vi "Init Hardware.vi"(8 "error in (no error)":errorcluster, 11 "Tektronix Driver in":refnum<class "Tektronix 4000 Driver.lvclass">) -> (0 "error out":errorcluster, 3 "Tektronix Driver out":refnum<class "Tektronix 4000 Driver.lvclass">)   [LabVIEW 2020, in "Tektronix 4000 Driver.lvclass"]
uses:
  Tektronix 4000 Driver.lvclass
  C:/GitHub/NHMFL_Core/Libraries/Instruments/Tektronix/Tektronix Driver/Tektronix Driver.lvclass
  <instrlib>/Tektronix DPO MSO 2000 4000 Series/Tektronix DPO MSO 2000 4000 Series.lvlib
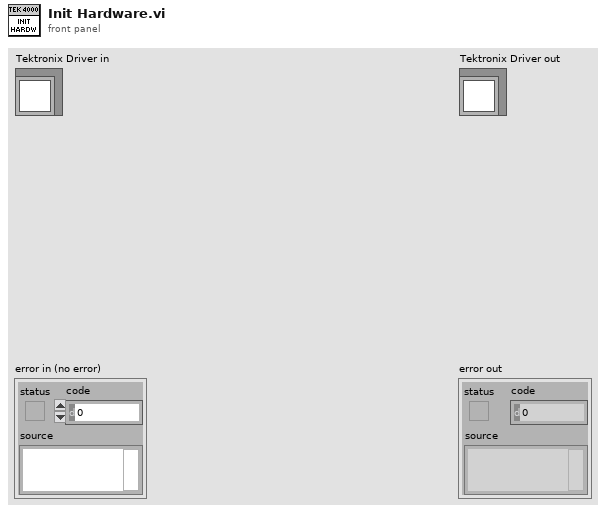
[diagram p1: front panel]
types:
  T1 = typedef "Tektronix Configuration.ctl" = cluster{"Channel":i32, "Number of averages":i32, "Input impedace":enum16{"1 M Ohm", "50 Ohm"}, "Vertical coupling":enum16{"AC", "DC", "Ground"}}
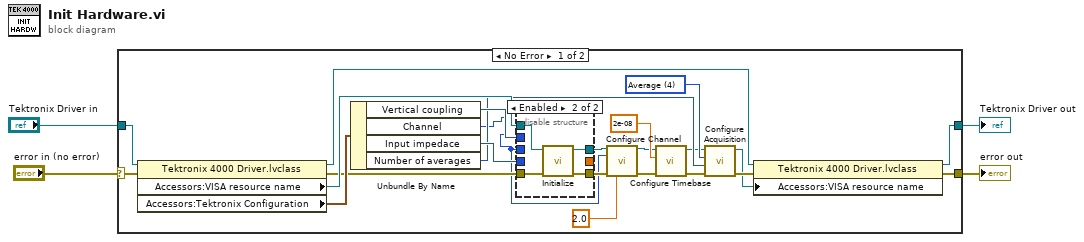
[diagram p0: block diagram]
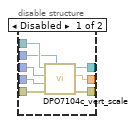
[diagram p2: hidden frame]
diagram:
  n1 = case shown="No Error" "error in (no error)" {
    selector: "error in (no error)" -> [w27 w41]
    tunnel: [w20 w41] -> w3
    tunnel: [w18 w40] -> w1
    tunnel: "Tektronix Driver in" -> [w26 w40]
    frame No Error {
      w17 = u16 4 items=["Sample", "Peak Detect", "Hi Res", "Envelope", "Average"] ("Acquisition Type (0: Sample)")
      n2 = property class="Tektronix 4000 Driver.lvclass"(reference=w26, error in=w27) -> (reference out=w19:refnum<class "Tektronix 4000 Driver.lvclass">, error out=w23:errorcluster, "Accessors:VISA resource name"=w25:refnum<visa-resource-name>, "Accessors:Tektronix Configuration"=w24:T1)
      n3 = Unbundle By Name(w24) -> ("Vertical coupling"=w22:enum16{"AC", "DC", "Ground"}, "Channel"=w6:i32, "Input impedace"=w21:enum16{"1 M Ohm", "50 Ohm"}, "Number of averages"=w16:i32)
      n4 = disable-structure shown="Enabled" {
        disable-tunnel: w25 -> [w35 w39]
        disable-tunnel: w23 -> [w34 w38]
        disable-tunnel: w22 -> [w33 _]
        disable-tunnel: [w32 _] -> _
        disable-tunnel: [w31 w36] -> w7
        disable-tunnel: [w30 w37] -> w10
        disable-tunnel: w6 -> [w29 _]
        disable-tunnel: w21 -> [w28 _]
        frame Disabled {
          n5 = call "DPO7104c_vert_scale.vi"("Vertical Coupling (1: DC)"=w33, "error in (no error)"=w34, "Input Impedance (0: 1M ohm)"=w28, "Channel (0: Channel 1)"=w29, "VISA resource name"=w35) -> ("error out"=w31:errorcluster, "vertical range"=w32:dbl, "VISA resource name out"=w30:refnum<visa-resource-name>)  [unwired: 4 in]
        }
        frame Enabled {
          n6 = call <instrlib>:"Initialize.vi"("error in (no error)"=w38, "VISA resource name"=w39) -> ("error out"=w36:errorcluster, "VISA resource name out"=w37:refnum<visa-resource-name>)  [unwired: 8 in]
        }
      }
      n7 = call <instrlib>:"Configure Channel.vi"("VISA resource name"=w10, "Channel (0: Channel 1)"=w6, "error in (no error)"=w7, "Vertical Range (10.0 V)"=2.0) -> ("VISA resource name out"=w9:refnum<visa-resource-name>, "error out"=w8:errorcluster)  [unwired: 10 in]
      n8 = call <instrlib>:"Configure Timebase.vi"("error in (no error)"=w8, "Timebase (0.0005 s)"=2e-08, "VISA resource name"=w9) -> ("error out"=w12:errorcluster, "VISA resource name out"=w13:refnum<visa-resource-name>)  [unwired: 7 in]
      n9 = call <instrlib>:"Configure Acquisition.vi"("error in (no error)"=w12, "Number of Waveform Acquisitions (16)"=w16, "Acquisition Type (0: Sample)"=w17, "VISA resource name"=w13) -> ("error out"=w15:errorcluster, "VISA resource name out"=w14:refnum<visa-resource-name>)  [unwired: 6 in]
      n10 = property class="Tektronix 4000 Driver.lvclass"(reference=w19, error in=w15, "Accessors:VISA resource name"=w14) -> (reference out=w18:refnum<class "Tektronix 4000 Driver.lvclass">, error out=w20:errorcluster)
    }
    frame Error {
    }
  }
  "error out" <- w3
  "Tektronix Driver out" <- w1
